vi "Generate Pulse Train.vi"() -> ()   [LabVIEW 2021]
panel:
  in  "Num pulses":i32
  in  "Duty Cycle":dbl
  in  "Frequency (Hz)":dbl
  in  "device name":tag="Dev1"
  in  "Start":bool
  in  "stop":bool
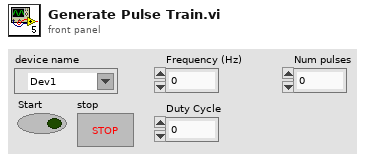
[diagram p1: front panel]
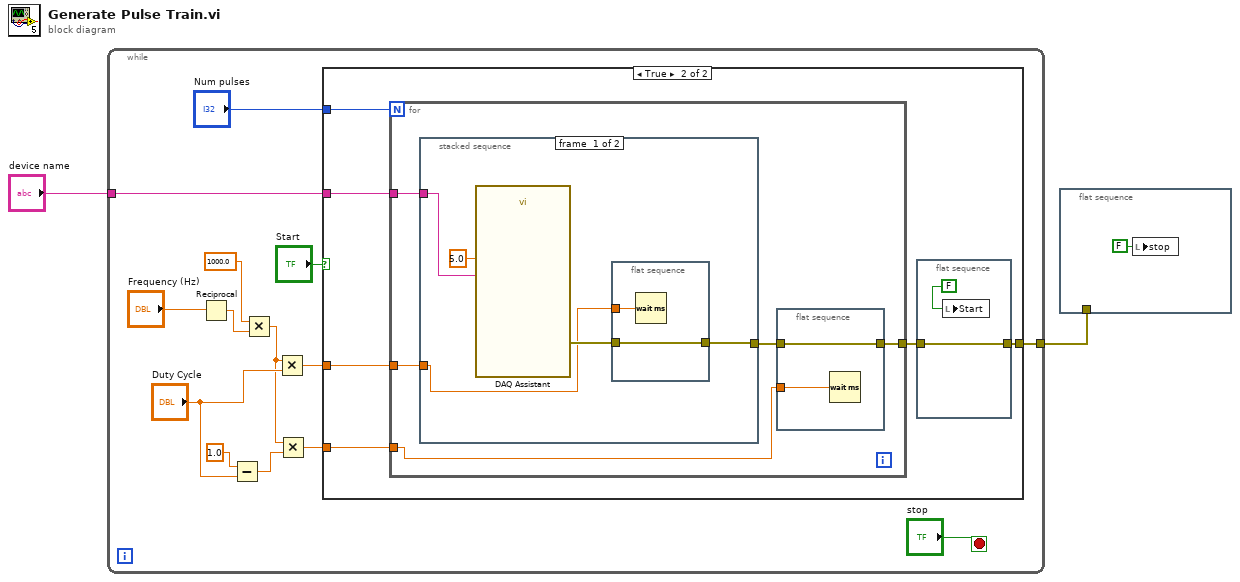
[diagram p0: block diagram]
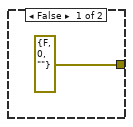
[diagram p2: hidden frame]
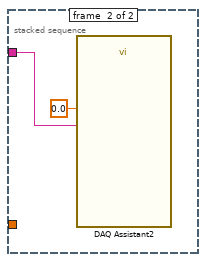
[diagram p3: hidden frame]
diagram:
  n1 = while {
    tunnel: "device name" -> [w16]
    tunnel: [w14] -> w1
    stop <- "stop" stop-if-true
    n2 = Reciprocal(x="Frequency (Hz)") -> (1/x=w5:dbl)
    n3 = Subtract(x=1.0, y="Duty Cycle") -> (x-y=w12:dbl)
    n4 = Multiply(x=1000.0, y=w5) -> (x*y=w4:dbl)
    n5 = Multiply(x=w4, y="Duty Cycle") -> (x*y=w7:dbl)
    n6 = Multiply(x=w4, y=w12) -> (x*y=w8:dbl)
    n7 = case shown="True" "Start" {
      tunnel: w16 -> [_ w23]
      tunnel: [errorcluster {"status"=FALSE, "code"=0, "source"=""} ("error out") w22] -> w14
      tunnel: w7 -> [_ w20]
      tunnel: w8 -> [_ w19]
      tunnel: "Num pulses" -> [_ w18]
      frame False {
      }
      frame True {
        n8 = for {
          N: w18 -> [_]
          tunnel: w23 -> [w30]
          tunnel: [w28] -> w21
          tunnel: w20 -> [w27]
          tunnel: w19 -> [w26]
          n9 = stacked-sequence {
            tunnel: w30 -> [w37 w41]
            tunnel: [w35 _] -> w29
            tunnel: w27 -> [w33 _]
            frame #0 {
              n10 = call "DAQ Assistant"("data"=5.0, "device name"=w37) -> ("error out"=w34:errorcluster)  [unwired: 16 in, 1 out]
              n11 = flat-sequence {
                tunnel: [w39] -> w35
                tunnel: w34 -> [w39]
                tunnel: w33 -> [w38]
                frame #0 {
                  n12 = Wait (ms)(milliseconds to wait=w38) -> ()  [unwired: 1 out]
                }
              }
            }
            frame #1 {
              n13 = call "DAQ Assistant2"("data"=0.0, "device name"=w41) -> ()  [unwired: 16 in, 2 out]
            }
          }
          n14 = flat-sequence {
            tunnel: w29 -> [w32]
            tunnel: [w32] -> w28
            tunnel: w26 -> [w31]
            frame #0 {
              n15 = Wait (ms)(milliseconds to wait=w31) -> ()  [unwired: 1 out]
            }
          }
        }
        n16 = flat-sequence {
          tunnel: [w25] -> w22
          tunnel: w21 -> [w25]
          frame #0 {
            n17 = local write "Start"(FALSE ("Sample")) -> ()
          }
        }
      }
    }
  }
  n18 = flat-sequence {
    tunnel: w1 -> [_]
    frame #0 {
      n19 = local write "stop"(FALSE ("stop")) -> ()
    }
  }
